vi "init_hw.vi"(8 "error in (no error)":errorcluster, 11 "smc100 in":refnum<class "smc100.lvclass">) -> (0 "error out":errorcluster, 2 "Boolean":bool=TRUE, 3 "smc100 out":refnum<class "smc100.lvclass">)   [LabVIEW 2019, in "smc100.lvlib" / "smc100.lvclass"]
uses:
  smc100.lvclass
  smc100.lvclass/smc100.ctl
  Read COM port.vi
  Write VISA Handle.vi
  <userlib>/SMC100 Controller_Drivers/SMC100.llb/enter / leave configuration state.vi
  <userlib>/SMC100 Controller_Drivers/SMC100.llb/enter / leave disable state.vi
panel:
  out "Controller's error":string
  out "Controller's state":string
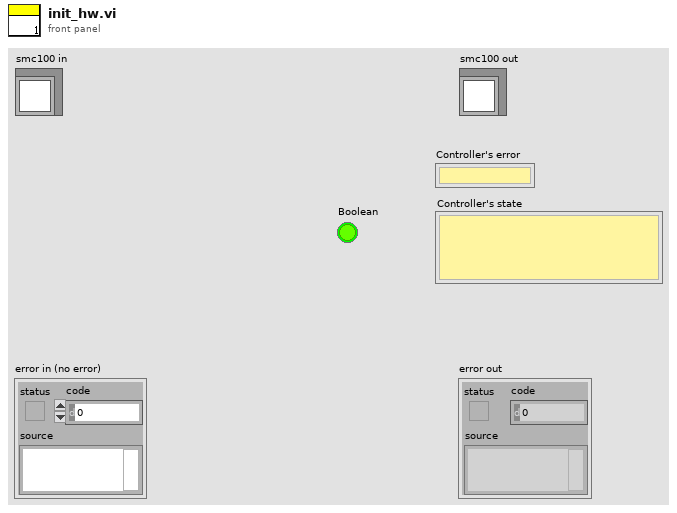
[diagram p1: front panel]
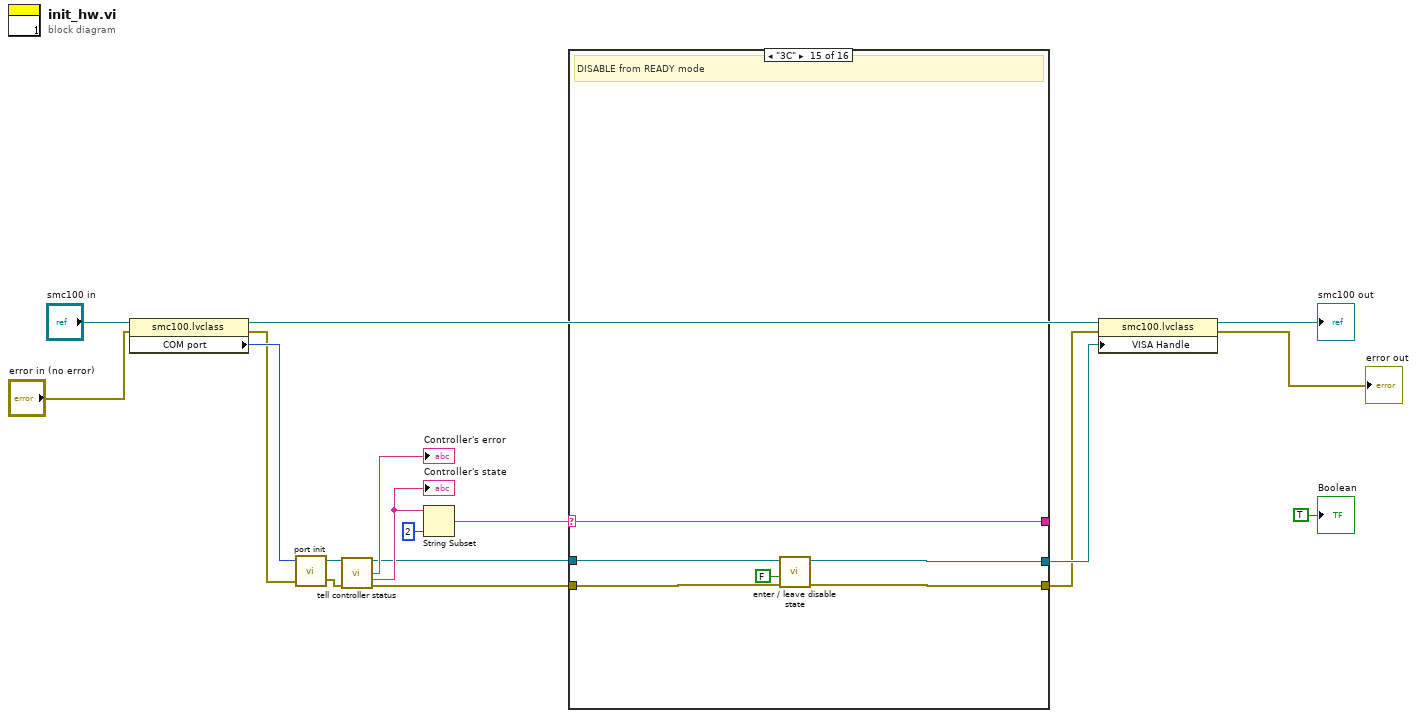
[diagram p0: block diagram]
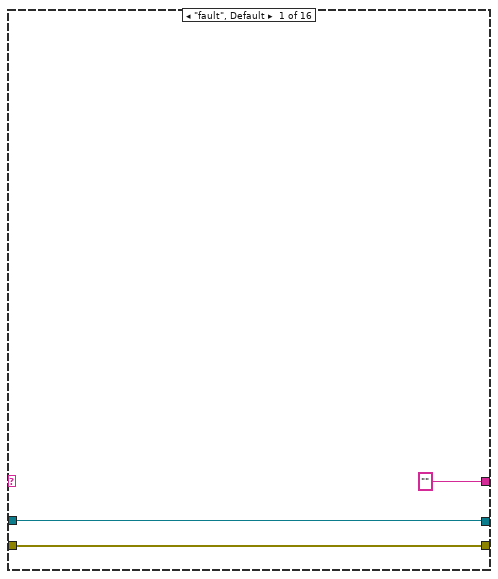
[diagram p2: hidden frame]
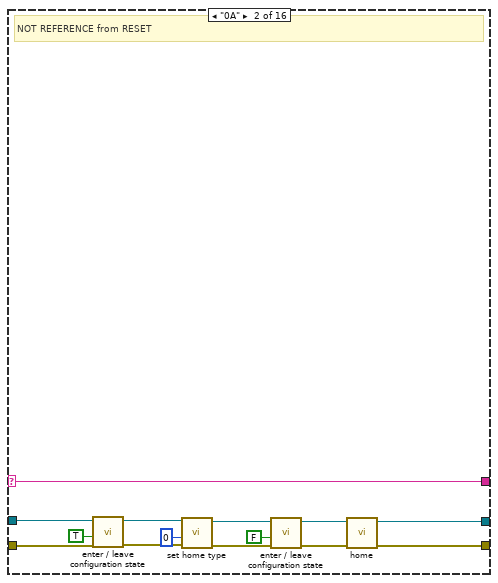
[diagram p3: hidden frame]
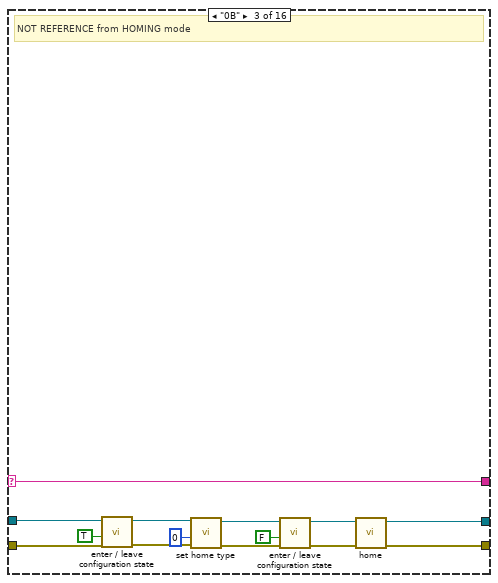
[diagram p4: hidden frame]
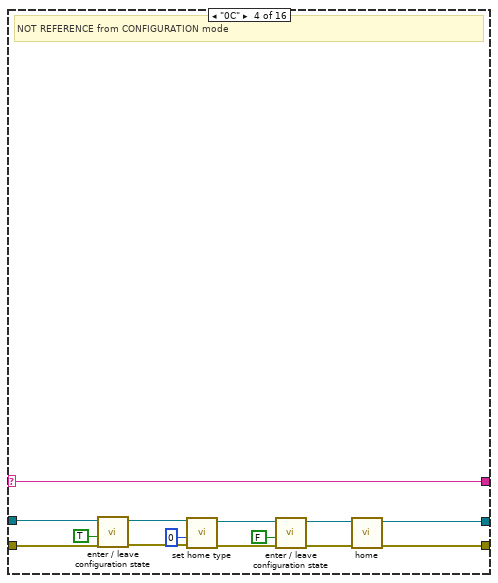
[diagram p5: hidden frame]
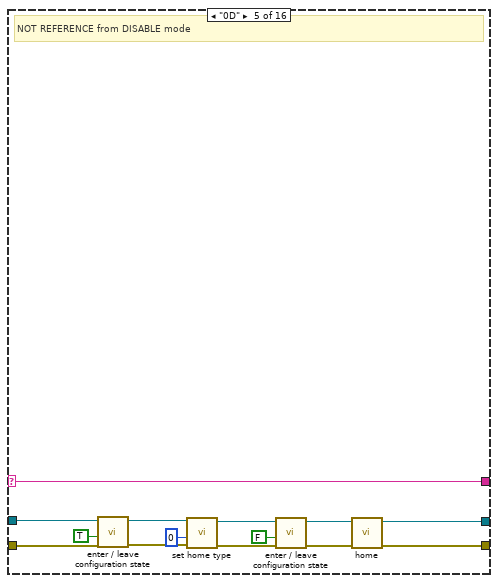
[diagram p6: hidden frame]
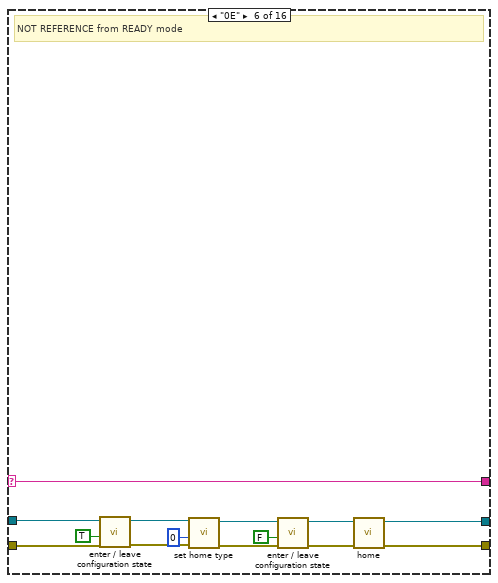
[diagram p7: hidden frame]
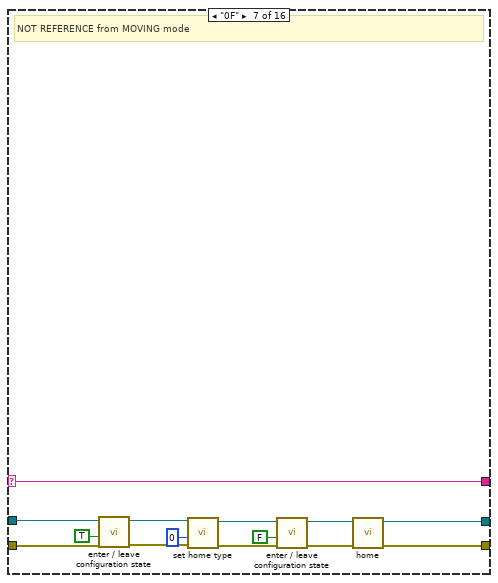
[diagram p8: hidden frame]
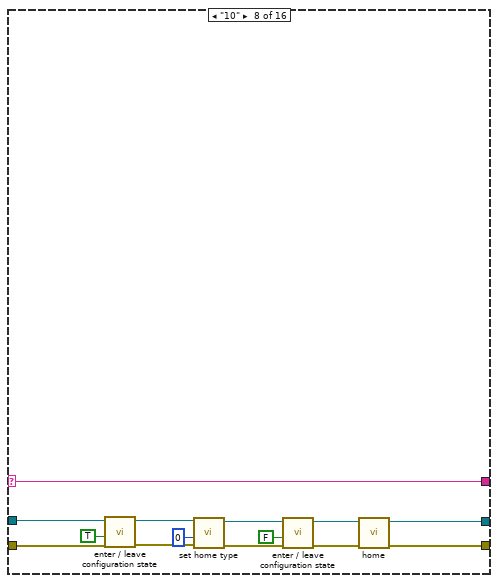
[diagram p9: hidden frame]
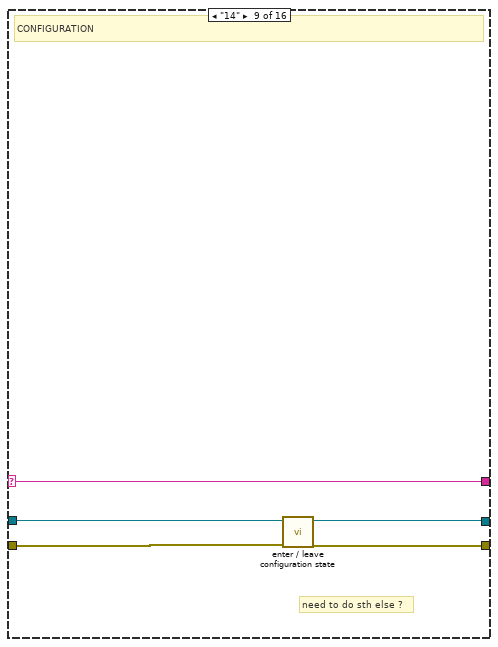
[diagram p10: hidden frame]
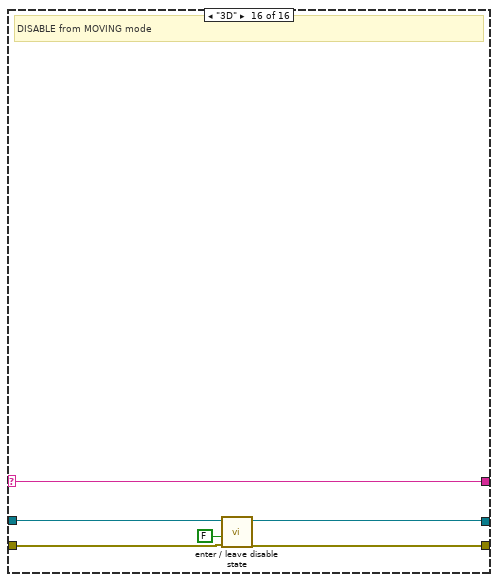
[diagram p16: hidden frame]
diagram:
  n1 = property class="smc100.lvclass"(reference="smc100 in", error in="error in (no error)") -> (reference out=w5:refnum<class "smc100.lvclass">, error out=w7:errorcluster, "COM port"=w8:u8)
  n2 = call <userlib>:"port init.vi"("error in"=w7, "SerialPort"=w8) -> ("error out"=w16:errorcluster, "Visa Handle"=w11:refnum<visa-resource-name>)  [unwired: 2 in]
  n3 = call <userlib>:"tell controller status.vi"("VISA Handle in"=w11, "error in"=w16) -> ("VISA Handle out"=w10:refnum<visa-resource-name>, "Controller's error"=→"Controller's error":string, "Controller's state"=w14:string, "error out"=w9:errorcluster)  [unwired: 8 in, 2 out]
  "Controller's state" <- w14
  n4 = String Subset(string=w14, length (rest)=2 ("length (rest)")) -> (substring=w12:string)  [unwired: 1 in]
  n5 = case shown="\"3C\"" w12 {
    selector: w12 -> [_ w35 w49 w63 w77 w91 w105 w119 w124 w127 w130 w133 w136 w139 w145 w151]
    tunnel: ["" w35 w49 w63 w77 w91 w105 w119 w124 w127 w130 w133 w136 w139 w145 w151] -> _
    tunnel: w10 -> [w20 w25 w36 w51 w67 w81 w95 w109 w123 w126 w129 w132 w135 w138 w144 w149]
    tunnel: w9 -> [w19 w24 w37 w50 w66 w80 w94 w108 w122 w125 w128 w131 w134 w137 w143 w148]
    tunnel: [w20 w23 w39 w53 w65 w79 w93 w107 w121 w126 w129 w132 w135 w138 w142 w147] -> w3
    tunnel: [w19 w22 w38 w52 w64 w78 w92 w106 w120 w125 w128 w131 w134 w137 w141 w146] -> w2
    frame "fault", Default {
    }
    frame "0A" {
      # "NOT REFERENCE from RESET"
      n6 = call "enter / leave configuration state.vi"("error in"=w24, "enter configuration state (True)"=TRUE, "VISA handle in"=w25) -> ("error out"=w29:errorcluster, "VISA handle out"=w31:refnum<visa-resource-name>)  [unwired: 5 in, 2 out]
      n7 = call <userlib>:"set home type.vi"("error in"=w29, "Home type value :\n0 use MZ switch and encoder Index\n1 use current position as HOME\n2 use MZ switch only\n3 use EoR- switch and encoder Index\n4 use EoR- switch only"=0 ("Home type value :\n0 use MZ switch and encoder Index\n1 use current position as HOME\n2 use MZ switch only\n3 use EoR- switch and encoder Index\n4 use EoR- switch only"), "VISA Handle in"=w31) -> ("error out"=w30:errorcluster, "VISA Handle out"=w32:refnum<visa-resource-name>)  [unwired: 3 in, 2 out]
      n8 = call "enter / leave configuration state.vi"("error in"=w30, "enter configuration state (True)"=FALSE, "VISA handle in"=w32) -> ("error out"=w34:errorcluster, "VISA handle out"=w33:refnum<visa-resource-name>)  [unwired: 5 in, 2 out]
      n9 = call <userlib>:"home.vi"("error in"=w34, "VISA Handle in"=w33) -> ("error out"=w22:errorcluster, "VISA Handle out"=w23:refnum<visa-resource-name>)  [unwired: 4 in, 2 out]
    }
    frame "0B" {
      # "NOT REFERENCE from HOMING mode"
      n10 = call "enter / leave configuration state.vi"("error in"=w37, "enter configuration state (True)"=TRUE, "VISA handle in"=w36) -> ("error out"=w48:errorcluster, "VISA handle out"=w46:refnum<visa-resource-name>)  [unwired: 5 in, 2 out]
      n11 = call <userlib>:"set home type.vi"("error in"=w48, "Home type value :\n0 use MZ switch and encoder Index\n1 use current position as HOME\n2 use MZ switch only\n3 use EoR- switch and encoder Index\n4 use EoR- switch only"=0 ("Home type value :\n0 use MZ switch and encoder Index\n1 use current position as HOME\n2 use MZ switch only\n3 use EoR- switch and encoder Index\n4 use EoR- switch only"), "VISA Handle in"=w46) -> ("error out"=w47:errorcluster, "VISA Handle out"=w45:refnum<visa-resource-name>)  [unwired: 3 in, 2 out]
      n12 = call "enter / leave configuration state.vi"("error in"=w47, "enter configuration state (True)"=FALSE, "VISA handle in"=w45) -> ("error out"=w43:errorcluster, "VISA handle out"=w44:refnum<visa-resource-name>)  [unwired: 5 in, 2 out]
      n13 = call <userlib>:"home.vi"("error in"=w43, "VISA Handle in"=w44) -> ("error out"=w38:errorcluster, "VISA Handle out"=w39:refnum<visa-resource-name>)  [unwired: 4 in, 2 out]
    }
    frame "0C" {
      # "NOT REFERENCE from CONFIGURATION mode"
      n14 = call "enter / leave configuration state.vi"("error in"=w50, "enter configuration state (True)"=TRUE, "VISA handle in"=w51) -> ("error out"=w57:errorcluster, "VISA handle out"=w59:refnum<visa-resource-name>)  [unwired: 5 in, 2 out]
      n15 = call <userlib>:"set home type.vi"("error in"=w57, "Home type value :\n0 use MZ switch and encoder Index\n1 use current position as HOME\n2 use MZ switch only\n3 use EoR- switch and encoder Index\n4 use EoR- switch only"=0 ("Home type value :\n0 use MZ switch and encoder Index\n1 use current position as HOME\n2 use MZ switch only\n3 use EoR- switch and encoder Index\n4 use EoR- switch only"), "VISA Handle in"=w59) -> ("error out"=w58:errorcluster, "VISA Handle out"=w60:refnum<visa-resource-name>)  [unwired: 3 in, 2 out]
      n16 = call "enter / leave configuration state.vi"("error in"=w58, "enter configuration state (True)"=FALSE, "VISA handle in"=w60) -> ("error out"=w62:errorcluster, "VISA handle out"=w61:refnum<visa-resource-name>)  [unwired: 5 in, 2 out]
      n17 = call <userlib>:"home.vi"("error in"=w62, "VISA Handle in"=w61) -> ("error out"=w52:errorcluster, "VISA Handle out"=w53:refnum<visa-resource-name>)  [unwired: 4 in, 2 out]
    }
    frame "0D" {
      # "NOT REFERENCE from DISABLE mode"
      n18 = call "enter / leave configuration state.vi"("error in"=w66, "enter configuration state (True)"=TRUE, "VISA handle in"=w67) -> ("error out"=w71:errorcluster, "VISA handle out"=w73:refnum<visa-resource-name>)  [unwired: 5 in, 2 out]
      n19 = call <userlib>:"set home type.vi"("error in"=w71, "Home type value :\n0 use MZ switch and encoder Index\n1 use current position as HOME\n2 use MZ switch only\n3 use EoR- switch and encoder Index\n4 use EoR- switch only"=0 ("Home type value :\n0 use MZ switch and encoder Index\n1 use current position as HOME\n2 use MZ switch only\n3 use EoR- switch and encoder Index\n4 use EoR- switch only"), "VISA Handle in"=w73) -> ("error out"=w72:errorcluster, "VISA Handle out"=w74:refnum<visa-resource-name>)  [unwired: 3 in, 2 out]
      n20 = call "enter / leave configuration state.vi"("error in"=w72, "enter configuration state (True)"=FALSE, "VISA handle in"=w74) -> ("error out"=w76:errorcluster, "VISA handle out"=w75:refnum<visa-resource-name>)  [unwired: 5 in, 2 out]
      n21 = call <userlib>:"home.vi"("error in"=w76, "VISA Handle in"=w75) -> ("error out"=w64:errorcluster, "VISA Handle out"=w65:refnum<visa-resource-name>)  [unwired: 4 in, 2 out]
    }
    frame "0E" {
      # "NOT REFERENCE from READY mode"
      n22 = call "enter / leave configuration state.vi"("error in"=w80, "enter configuration state (True)"=TRUE, "VISA handle in"=w81) -> ("error out"=w85:errorcluster, "VISA handle out"=w87:refnum<visa-resource-name>)  [unwired: 5 in, 2 out]
      n23 = call <userlib>:"set home type.vi"("error in"=w85, "Home type value :\n0 use MZ switch and encoder Index\n1 use current position as HOME\n2 use MZ switch only\n3 use EoR- switch and encoder Index\n4 use EoR- switch only"=0 ("Home type value :\n0 use MZ switch and encoder Index\n1 use current position as HOME\n2 use MZ switch only\n3 use EoR- switch and encoder Index\n4 use EoR- switch only"), "VISA Handle in"=w87) -> ("error out"=w86:errorcluster, "VISA Handle out"=w88:refnum<visa-resource-name>)  [unwired: 3 in, 2 out]
      n24 = call "enter / leave configuration state.vi"("error in"=w86, "enter configuration state (True)"=FALSE, "VISA handle in"=w88) -> ("error out"=w90:errorcluster, "VISA handle out"=w89:refnum<visa-resource-name>)  [unwired: 5 in, 2 out]
      n25 = call <userlib>:"home.vi"("error in"=w90, "VISA Handle in"=w89) -> ("error out"=w78:errorcluster, "VISA Handle out"=w79:refnum<visa-resource-name>)  [unwired: 4 in, 2 out]
    }
    frame "0F" {
      # "NOT REFERENCE from MOVING mode"
      n26 = call "enter / leave configuration state.vi"("error in"=w94, "enter configuration state (True)"=TRUE, "VISA handle in"=w95) -> ("error out"=w99:errorcluster, "VISA handle out"=w101:refnum<visa-resource-name>)  [unwired: 5 in, 2 out]
      n27 = call <userlib>:"set home type.vi"("error in"=w99, "Home type value :\n0 use MZ switch and encoder Index\n1 use current position as HOME\n2 use MZ switch only\n3 use EoR- switch and encoder Index\n4 use EoR- switch only"=0 ("Home type value :\n0 use MZ switch and encoder Index\n1 use current position as HOME\n2 use MZ switch only\n3 use EoR- switch and encoder Index\n4 use EoR- switch only"), "VISA Handle in"=w101) -> ("error out"=w100:errorcluster, "VISA Handle out"=w102:refnum<visa-resource-name>)  [unwired: 3 in, 2 out]
      n28 = call "enter / leave configuration state.vi"("error in"=w100, "enter configuration state (True)"=FALSE, "VISA handle in"=w102) -> ("error out"=w104:errorcluster, "VISA handle out"=w103:refnum<visa-resource-name>)  [unwired: 5 in, 2 out]
      n29 = call <userlib>:"home.vi"("error in"=w104, "VISA Handle in"=w103) -> ("error out"=w92:errorcluster, "VISA Handle out"=w93:refnum<visa-resource-name>)  [unwired: 4 in, 2 out]
    }
    frame "10" {
      n30 = call "enter / leave configuration state.vi"("error in"=w108, "enter configuration state (True)"=TRUE, "VISA handle in"=w109) -> ("error out"=w113:errorcluster, "VISA handle out"=w115:refnum<visa-resource-name>)  [unwired: 5 in, 2 out]
      n31 = call <userlib>:"set home type.vi"("error in"=w113, "Home type value :\n0 use MZ switch and encoder Index\n1 use current position as HOME\n2 use MZ switch only\n3 use EoR- switch and encoder Index\n4 use EoR- switch only"=0 ("Home type value :\n0 use MZ switch and encoder Index\n1 use current position as HOME\n2 use MZ switch only\n3 use EoR- switch and encoder Index\n4 use EoR- switch only"), "VISA Handle in"=w115) -> ("error out"=w114:errorcluster, "VISA Handle out"=w116:refnum<visa-resource-name>)  [unwired: 3 in, 2 out]
      n32 = call "enter / leave configuration state.vi"("error in"=w114, "enter configuration state (True)"=FALSE, "VISA handle in"=w116) -> ("error out"=w118:errorcluster, "VISA handle out"=w117:refnum<visa-resource-name>)  [unwired: 5 in, 2 out]
      n33 = call <userlib>:"home.vi"("error in"=w118, "VISA Handle in"=w117) -> ("error out"=w106:errorcluster, "VISA Handle out"=w107:refnum<visa-resource-name>)  [unwired: 4 in, 2 out]
    }
    frame "14" {
      # "need to do sth else ?"
      # "CONFIGURATION"
      n34 = call "enter / leave configuration state.vi"("error in"=w122, "VISA handle in"=w123) -> ("error out"=w120:errorcluster, "VISA handle out"=w121:refnum<visa-resource-name>)  [unwired: 6 in, 2 out]
    }
    frame "1E" {
      # "HOMING"
    }
    frame "28" {
      # "MOVING"
    }
    frame "32" {
      # "READY from HOMING mode"
    }
    frame "33" {
      # "READY from MOVING mode"
    }
    frame "34" {
      # "READY from DISABLE mode"
    }
    frame "3C" {
      # "DISABLE from READY mode"
      n35 = call "enter / leave disable state.vi"("error in"=w143, "enter disable state (True)"=FALSE, "VISA handle in"=w144) -> ("error out"=w141:errorcluster, "VISA handle out"=w142:refnum<visa-resource-name>)  [unwired: 5 in, 2 out]
    }
    frame "3D" {
      # "DISABLE from MOVING mode"
      n36 = call "enter / leave disable state.vi"("error in"=w148, "enter disable state (True)"=FALSE, "VISA handle in"=w149) -> ("error out"=w146:errorcluster, "VISA handle out"=w147:refnum<visa-resource-name>)  [unwired: 5 in, 2 out]
    }
  }
  n37 = property class="smc100.lvclass"(reference=w5, error in=w2, "VISA Handle"=w3) -> (reference out=→"smc100 out":refnum<class "smc100.lvclass">, error out=→"error out":errorcluster)
  "Boolean" <- TRUE ("Boolean")
